vi "Constructor.vi"(8 "error in (no error)":errorcluster, 11 "Reggiano in":refnum<class "Reggiano.lvclass">) -> (0 "error out":errorcluster, 2 "Ingredients":string, 3 "Reggiano out":refnum<class "Reggiano.lvclass">)   [LabVIEW 2013, in "Reggiano.lvclass"]
uses:
  Reggiano.lvclass
panel:
  # "§Ú¬O¨Å¹T°_¥q"
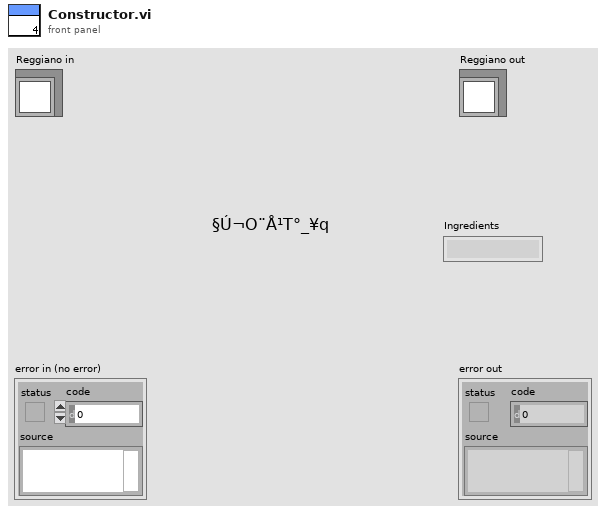
[diagram p1: front panel]
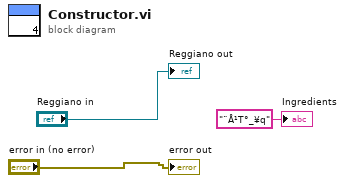
[diagram p0: block diagram]
diagram:
  "error out" <- "error in (no error)"
  "Reggiano out" <- "Reggiano in"
  "Ingredients" <- "¨Å¹T°_¥q" ("Ingredients")
